vi "Notify PV Monitoring.vi"(8 "Error In":errorcluster, 11 "BNT_SLTagMonitor in":refnum<class "BNT_SLTagMonitor.lvclass">) -> (0 "Error Out":errorcluster, 3 "BNT_SLTagMonitor out":refnum<class "BNT_SLTagMonitor.lvclass">)   [LabVIEW 2019, in "BNT_SLTagMonitor.lvlib" / "BNT_SLTagMonitor.lvclass"]
doc: "Notify PV readout."
uses:
  BNT_SLTagMonitor.lvclass
  CSPP_Core/Actors/CSPP_PVMonitor/CSPP_PVMonitor.lvclass
  C:/Users/Holger/Documents/LVP/CSPP/CSPP-Template/Packages/CSPP_Core/Actors/CSPP_PVMonitor/CSPP_PVMonitor.lvclass
  C:/Users/Holger/Documents/LVP/CSPP/CSPP-Template/Packages/CSPP_Core/Actors/CSPP_BaseActor/CSPP_BaseActor.lvclass
  C:/Program Files (x86)/National Instruments/LabVIEW 2019/vi.lib/ActorFramework/Actor/Actor.lvclass
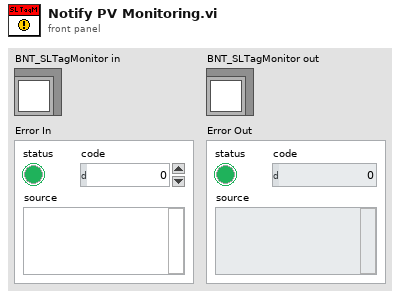
[diagram p1: front panel]
types:
  T1 = cluster{"PV URL":string, "Observers":cluster{"Enqueuer":refnum<class "Message Enqueuer.lvclass">, "CSPP_PVUpdate Msg":refnum<class "CSPP_PVUpdate Msg.lvclass">}[]}[]
  T2 = cluster{"SL Tags":refnum<class "NI Skyline Tag.lvclass">[], "PV Connections":cluster{"PV URL":string, "Observers":cluster{"Enqueuer":refnum<class "Message Enqueuer.lvclass">, "CSPP_PVUpdate Msg":refnum<class "CSPP_PVUpdate Msg.lvclass">}[]}[]}
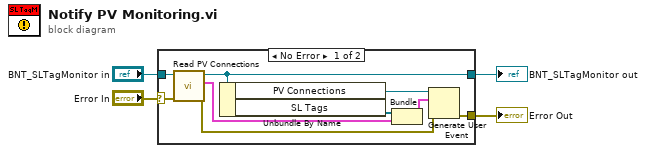
[diagram p0: block diagram]
diagram:
  n1 = case shown="No Error" "Error In" {
    selector: "Error In" -> [w12 w14]
    tunnel: "BNT_SLTagMonitor in" -> [w13 w15]
    tunnel: [w9 w15] -> w3
    tunnel: [w5 w14] -> w2
    frame No Error {
      n2 = call "Read PV Connections.vi"("error in (no error)"=w12, "CSPP_PVMonitor in"=w13) -> ("error out"=w6:errorcluster, "PV Connections"=w10:T1, "CSPP_PVMonitor out"=w9:refnum<class "BNT_SLTagMonitor.lvclass">)  [unwired: 7 in]
      n3 = Unbundle By Name(w9) -> ("PV Connections"=w8:refnum<user-event>, "SL Tags"=w11:refnum<class "NI Skyline Tag.lvclass">[])
      n4 = Bundle("SL Tags"=w11, "PV Connections"=w10) -> (w7:T2)  [unwired: 1 in]
      n5 = Generate User Event(user event=w8, event data cluster=w7, error in=w6) -> (error out=w5:errorcluster)  [unwired: 1 in, 1 out]
    }
    frame Error {
    }
  }
  "BNT_SLTagMonitor out" <- w3
  "Error Out" <- w2
